vi "SI prefix.vi"(9 "Array":dbl[](array[numeric]), 10 "Numeric":dbl format="%#_8f", 11 "Unit":string) -> (1 "Scaled Array":dbl[](array[numeric]), 2 "Scaled Number":dbl, 3 "modified unit":string)   [LabVIEW 2015]
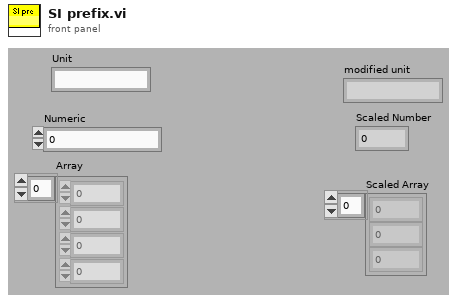
[diagram p1: front panel]
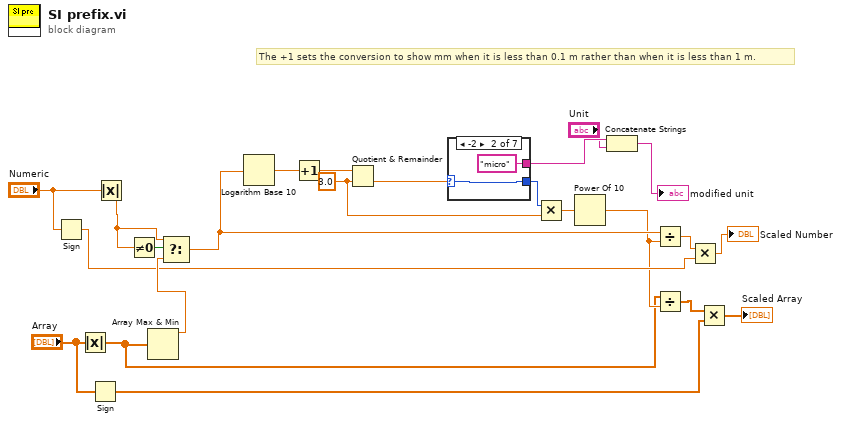
[diagram p0: block diagram]
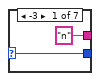
[diagram p2: hidden frame]
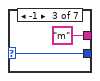
[diagram p3: hidden frame]
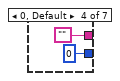
[diagram p4: hidden frame]
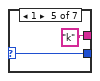
[diagram p5: hidden frame]
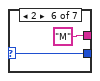
[diagram p6: hidden frame]
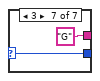
[diagram p7: hidden frame]
diagram:
  w21 = 3.0 ("y")
  # "The +1 sets the conversion to show mm when it is less than 0.1 m rather than when it is less than 1 m."
  n1 = Sign(1:"Numeric") -> (0:w9:dbl)
  n2 = Absolute Value(x="Array") -> (abs(x)=w3:dbl[])
  n3 = Sign(1:"Array") -> (0:w8:dbl[])
  n4 = Absolute Value(x="Numeric") -> (abs(x)=w13:dbl)
  n5 = Not Equal To 0?(x=w13) -> (x != 0?=w16:bool)
  n6 = Array Max & Min(array=w3) -> (max value=w14:dbl)  [unwired: 3 out]
  n7 = Select(t=w13, s=w16, f=w14) -> (s? t:f=w15:dbl)
  n8 = Logarithm Base 10(1:w15) -> (0:w23:dbl)
  n9 = Increment(x=w23) -> (x+1=w1:dbl)
  n10 = Quotient & Remainder(x=w1, y=w21) -> (floor(x/y)=w20:dbl)  [unwired: 1 out]
  n11 = case shown="-2" w20 {
    selector: w20 -> [w24 w27 w28 _ w32 w34 w36]
    tunnel: ["n" "micro" "m" "" "k" "M" "G"] -> w18
    tunnel: [w24 w27 w28 0 w32 w34 w36] -> w19
    frame -3 {
    }
    frame -2 {
    }
    frame -1 {
    }
    frame 0, Default {
    }
    frame 1 {
    }
    frame 2 {
    }
    frame 3 {
    }
  }
  n12 = Multiply(x=w19, y=w21) -> (x*y=w22:dbl)
  n13 = Power Of 10(x=w22) -> (10^x=w4:dbl)
  n14 = Concatenate Strings(w18, "Unit") -> (→"modified unit":string)
  n15 = Divide(x=w15, y=w4) -> (x/y=w6:dbl)
  n16 = Divide(x=w3, y=w4) -> (x/y=w5:dbl[])
  n17 = Multiply(x=w6, y=w9) -> (x*y=→"Scaled Number":dbl)
  n18 = Multiply(x=w5, y=w8) -> (x*y=→"Scaled Array":dbl[])
